vi "得出牌值.vi"(4 "牌4":dbl, 5 "牌3":dbl, 6 "牌2":dbl, 7 "牌1":dbl) -> (0 "牌4值":dbl, 1 "牌2值":dbl, 2 "牌3值":dbl, 3 "牌1值":dbl)   [LabVIEW 2014]
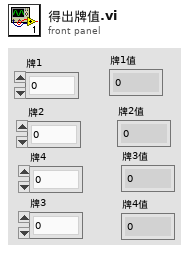
[diagram p1: front panel]
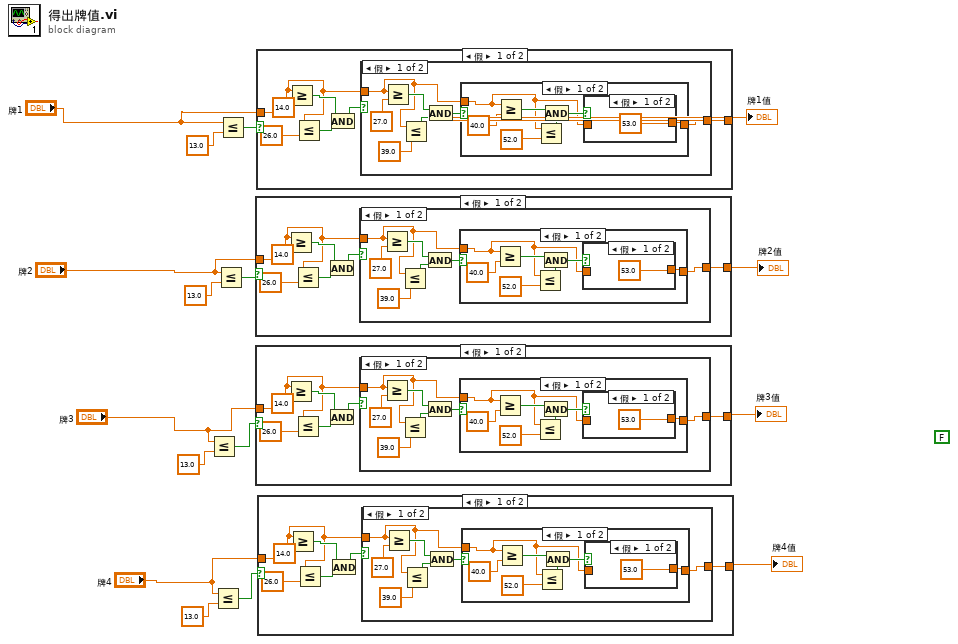
[diagram p0: block diagram]
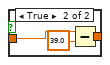
[diagram p2: hidden frame]
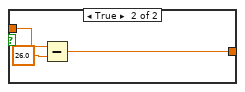
[diagram p3: hidden frame]
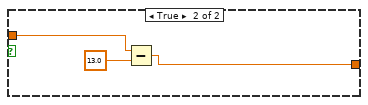
[diagram p4: hidden frame]
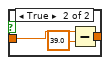
[diagram p6: hidden frame]
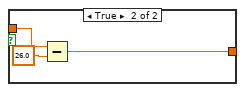
[diagram p7: hidden frame]
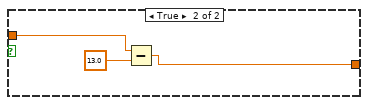
[diagram p8: hidden frame]
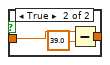
[diagram p10: hidden frame]
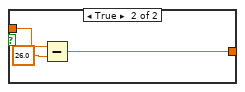
[diagram p11: hidden frame]
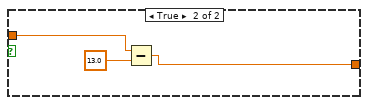
[diagram p12: hidden frame]
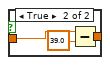
[diagram p14: hidden frame]
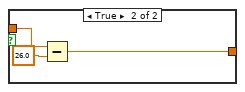
[diagram p15: hidden frame]
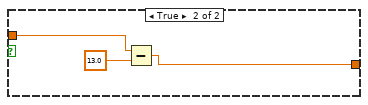
[diagram p16: hidden frame]
diagram:
  (unwired) FALSE
  n1 = Less Or Equal?(x="牌3", y=13.0) -> (x <= y?=w4:bool)
  n2 = Less Or Equal?(x="牌4", y=13.0) -> (x <= y?=w3:bool)
  n3 = Less Or Equal?(x="牌2", y=13.0) -> (x <= y?=w5:bool)
  n4 = Less Or Equal?(x="牌1", y=13.0) -> (x <= y?=w6:bool)
  n5 = case shown="假" w5 {
    tunnel: [w17 w48] -> w11
    tunnel: "牌2" -> [w18 w48]
    frame False {
      n6 = Greater Or Equal?(x=w18, y=14.0) -> (x >= y?=w20:bool)
      n7 = Less Or Equal?(x=w18, y=26.0) -> (x <= y?=w21:bool)
      n8 = And(x=w20, y=w21) -> (x .and. y?=w19:bool)
      n9 = case shown="假" w19 {
        tunnel: w18 -> [w25 w46]
        tunnel: [w24 w45] -> w17
        frame False {
          n10 = Greater Or Equal?(x=w25, y=27.0) -> (x >= y?=w28:bool)
          n11 = Less Or Equal?(x=w25, y=39.0) -> (x <= y?=w27:bool)
          n12 = And(x=w28, y=w27) -> (x .and. y?=w26:bool)
          n13 = case shown="假" w26 {
            tunnel: w25 -> [w33 w44]
            tunnel: [w32 w42] -> w24
            frame False {
              n14 = Greater Or Equal?(x=w33, y=40.0) -> (x >= y?=w35:bool)
              n15 = Less Or Equal?(x=w33, y=52.0) -> (x <= y?=w31:bool)
              n16 = And(x=w35, y=w31) -> (x .and. y?=w34:bool)
              n17 = case shown="假" w34 {
                tunnel: w33 -> [_ w40]
                tunnel: [53.0 ("y") w39] -> w32
                frame False {
                }
                frame True {
                  n18 = Subtract(x=w40, y=39.0) -> (x-y=w39:dbl)
                }
              }
            }
            frame True {
              n19 = Subtract(x=w44, y=26.0) -> (x-y=w42:dbl)
            }
          }
        }
        frame True {
          n20 = Subtract(x=w46, y=13.0) -> (x-y=w45:dbl)
        }
      }
    }
    frame True {
    }
  }
  "牌2值" <- w11
  n21 = case shown="假" w4 {
    tunnel: [w49 w80] -> w10
    tunnel: "牌3" -> [w50 w80]
    frame False {
      n22 = Greater Or Equal?(x=w50, y=14.0) -> (x >= y?=w52:bool)
      n23 = Less Or Equal?(x=w50, y=26.0) -> (x <= y?=w53:bool)
      n24 = And(x=w52, y=w53) -> (x .and. y?=w51:bool)
      n25 = case shown="假" w51 {
        tunnel: w50 -> [w57 w78]
        tunnel: [w56 w77] -> w49
        frame False {
          n26 = Greater Or Equal?(x=w57, y=27.0) -> (x >= y?=w60:bool)
          n27 = Less Or Equal?(x=w57, y=39.0) -> (x <= y?=w59:bool)
          n28 = And(x=w60, y=w59) -> (x .and. y?=w58:bool)
          n29 = case shown="假" w58 {
            tunnel: w57 -> [w65 w76]
            tunnel: [w64 w74] -> w56
            frame False {
              n30 = Greater Or Equal?(x=w65, y=40.0) -> (x >= y?=w67:bool)
              n31 = Less Or Equal?(x=w65, y=52.0) -> (x <= y?=w63:bool)
              n32 = And(x=w67, y=w63) -> (x .and. y?=w66:bool)
              n33 = case shown="假" w66 {
                tunnel: w65 -> [_ w72]
                tunnel: [53.0 ("y") w71] -> w64
                frame False {
                }
                frame True {
                  n34 = Subtract(x=w72, y=39.0) -> (x-y=w71:dbl)
                }
              }
            }
            frame True {
              n35 = Subtract(x=w76, y=26.0) -> (x-y=w74:dbl)
            }
          }
        }
        frame True {
          n36 = Subtract(x=w78, y=13.0) -> (x-y=w77:dbl)
        }
      }
    }
    frame True {
    }
  }
  "牌3值" <- w10
  n37 = case shown="假" w6 {
    tunnel: [w81 w112] -> w15
    tunnel: "牌1" -> [w82 w112]
    frame False {
      n38 = Greater Or Equal?(x=w82, y=14.0) -> (x >= y?=w84:bool)
      n39 = Less Or Equal?(x=w82, y=26.0) -> (x <= y?=w85:bool)
      n40 = And(x=w84, y=w85) -> (x .and. y?=w83:bool)
      n41 = case shown="假" w83 {
        tunnel: w82 -> [w89 w110]
        tunnel: [w88 w109] -> w81
        frame False {
          n42 = Greater Or Equal?(x=w89, y=27.0) -> (x >= y?=w92:bool)
          n43 = Less Or Equal?(x=w89, y=39.0) -> (x <= y?=w91:bool)
          n44 = And(x=w92, y=w91) -> (x .and. y?=w90:bool)
          n45 = case shown="假" w90 {
            tunnel: w89 -> [w97 w108]
            tunnel: [w96 w106] -> w88
            frame False {
              n46 = Greater Or Equal?(x=w97, y=40.0) -> (x >= y?=w99:bool)
              n47 = Less Or Equal?(x=w97, y=52.0) -> (x <= y?=w95:bool)
              n48 = And(x=w99, y=w95) -> (x .and. y?=w98:bool)
              n49 = case shown="假" w98 {
                tunnel: w97 -> [_ w104]
                tunnel: [53.0 ("y") w103] -> w96
                frame False {
                }
                frame True {
                  n50 = Subtract(x=w104, y=39.0) -> (x-y=w103:dbl)
                }
              }
            }
            frame True {
              n51 = Subtract(x=w108, y=26.0) -> (x-y=w106:dbl)
            }
          }
        }
        frame True {
          n52 = Subtract(x=w110, y=13.0) -> (x-y=w109:dbl)
        }
      }
    }
    frame True {
    }
  }
  "牌1值" <- w15
  n53 = case shown="假" w3 {
    tunnel: [w113 w144] -> w9
    tunnel: "牌4" -> [w114 w144]
    frame False {
      n54 = Greater Or Equal?(x=w114, y=14.0) -> (x >= y?=w116:bool)
      n55 = Less Or Equal?(x=w114, y=26.0) -> (x <= y?=w117:bool)
      n56 = And(x=w116, y=w117) -> (x .and. y?=w115:bool)
      n57 = case shown="假" w115 {
        tunnel: w114 -> [w121 w142]
        tunnel: [w120 w141] -> w113
        frame False {
          n58 = Greater Or Equal?(x=w121, y=27.0) -> (x >= y?=w124:bool)
          n59 = Less Or Equal?(x=w121, y=39.0) -> (x <= y?=w123:bool)
          n60 = And(x=w124, y=w123) -> (x .and. y?=w122:bool)
          n61 = case shown="假" w122 {
            tunnel: w121 -> [w129 w140]
            tunnel: [w128 w138] -> w120
            frame False {
              n62 = Greater Or Equal?(x=w129, y=40.0) -> (x >= y?=w131:bool)
              n63 = Less Or Equal?(x=w129, y=52.0) -> (x <= y?=w127:bool)
              n64 = And(x=w131, y=w127) -> (x .and. y?=w130:bool)
              n65 = case shown="假" w130 {
                tunnel: w129 -> [_ w136]
                tunnel: [53.0 ("y") w135] -> w128
                frame False {
                }
                frame True {
                  n66 = Subtract(x=w136, y=39.0) -> (x-y=w135:dbl)
                }
              }
            }
            frame True {
              n67 = Subtract(x=w140, y=26.0) -> (x-y=w138:dbl)
            }
          }
        }
        frame True {
          n68 = Subtract(x=w142, y=13.0) -> (x-y=w141:dbl)
        }
      }
    }
    frame True {
    }
  }
  "牌4值" <- w9
